vi "Rang wear off.vi"(8 "error in (no error)":errorcluster caption="错误输入（无错误）", 10 "字符串":string, 11 "Popup 输入":refnum<class "Popup.lvclass"> caption="DNL_LabVIEW Object in") -> (0 "error out":errorcluster caption="错误输出", 3 "Popup 输出":refnum<class "Popup.lvclass"> caption="DNL_LabVIEW Object out")   [LabVIEW 2017, in "Popup.lvclass"]
uses:
  Popup.lvclass
  Popup.lvclass/Popup.ctl
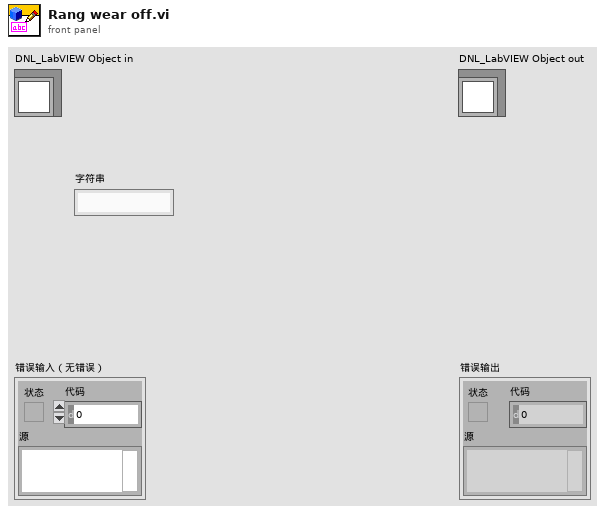
[diagram p1: front panel]
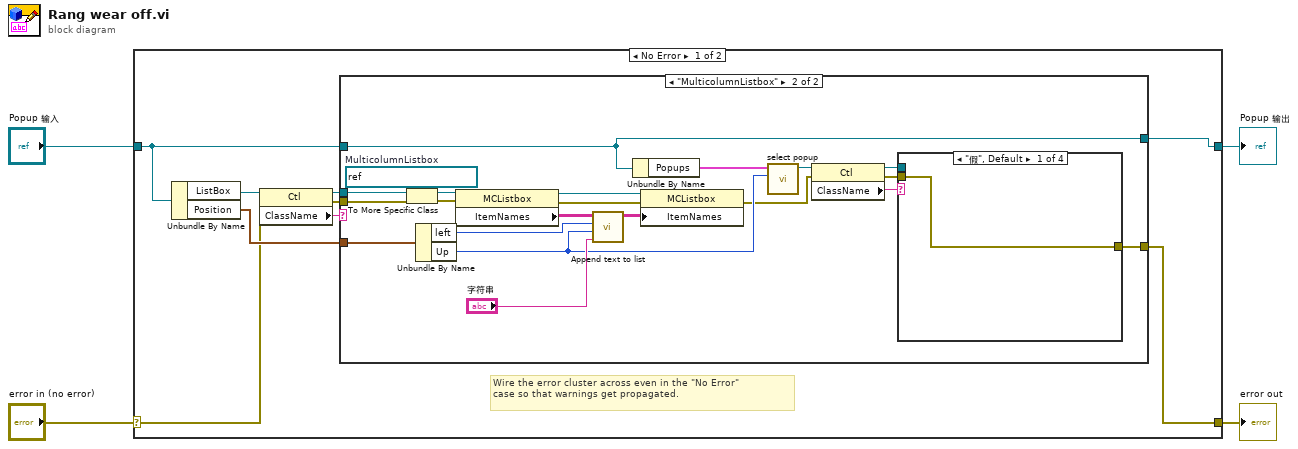
[diagram p0: block diagram]
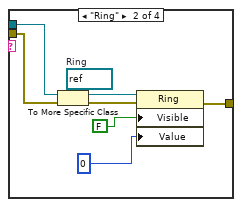
[diagram p3: hidden frame]
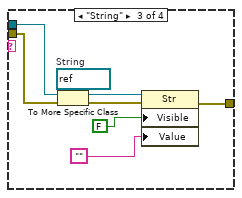
[diagram p4: hidden frame]
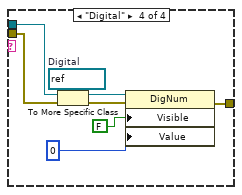
[diagram p5: hidden frame]
diagram:
  n1 = case shown="No Error" "error in (no error)" {
    selector: "error in (no error)" -> [w7 w63]
    tunnel: [w11 w63] -> w3
    tunnel: [w5 w62] -> w1
    tunnel: "Popup 输入" -> [w12 w62]
    frame No Error {
      # "Wire the error cluster across even in the \"No Error\"\ncase so that warnings get propagated."
      n2 = Unbundle By Name(w12) -> ("ListBox"=w10:refnum<vi>, "Position"=w13:cluster{"left":i32, "Up":i32})
      n3 = property class="Ctl"(reference=w10, error in=w7) -> (reference out=w9:refnum<vi>, error out=w8:errorcluster, "ClassName"=w6:string)
      n4 = case shown="\"MulticolumnListbox\"" w6 {
        tunnel: w13 -> [_ w33]
        tunnel: w12 -> [w14 w23]
        tunnel: [w15 w30] -> w11
        tunnel: w9 -> [_ w25]
        tunnel: w8 -> [w15 w24]
        tunnel: [w14 w23] -> w5
        frame "假", Default {
        }
        frame "MulticolumnListbox" {
          w36 = refnum<vi> refnum  # MulticolumnListbox
          n5 = To More Specific Class(target class=w36, reference=w25, error in=w24) -> (specific class reference=w35:refnum<vi>, error out=w34:errorcluster)
          n6 = Unbundle By Name(w33) -> ("left"=w27:i32, "Up"=w21:i32)
          n7 = property class="MCListbox"(reference=w35, error in=w34) -> (reference out=w32:refnum<vi>, error out=w31:errorcluster, "ItemNames"=w29:string[][])
          n8 = call "Append text to list.vi"("Text"="字符串", "Up"=w21, "Left"=w27, "List Text[]"=w29) -> ("List out[]"=w28:string[][])  [unwired: 7 in]
          n9 = Unbundle By Name(w23) -> ("Popups"=w22:cluster{"Referens":refnum<vi>, "Column":i32}[])
          n10 = property class="MCListbox"(reference=w32, error in=w31, "ItemNames"=w28) -> (error out=w19:errorcluster)  [unwired: 1 out]
          n11 = call "select popup.vi"("Column"=w21, "Popups"=w22) -> ("Ring输出"=w20:refnum<vi>)  [unwired: 9 in]
          n12 = property class="Ctl"(reference=w20, error in=w19) -> (reference out=w17:refnum<vi>, error out=w16:errorcluster, "ClassName"=w18:string)
          n13 = case shown="\"假\", Default" w18 {
            tunnel: [w37 w41 w49 w57] -> w30
            tunnel: w17 -> [_ w39 w48 w56]
            tunnel: w16 -> [w37 w38 w47 w55]
            frame "假", Default {
            }
            frame "Ring" {
              w45 = refnum<vi> refnum  # Ring
              n14 = To More Specific Class(target class=w45, reference=w39, error in=w38) -> (specific class reference=w44:refnum<vi>, error out=w43:errorcluster)
              n15 = property class="Ring"(reference=w44, error in=w43, "Visible"=FALSE, "Value"=u16 0) -> (error out=w41:errorcluster)  [unwired: 1 out]
            }
            frame "String" {
              w53 = refnum<vi> refnum  # String
              n16 = To More Specific Class(target class=w53, reference=w48, error in=w47) -> (specific class reference=w52:refnum<vi>, error out=w51:errorcluster)
              n17 = property class="Str"(reference=w52, error in=w51, "Visible"=FALSE, "Value"="") -> (error out=w49:errorcluster)  [unwired: 1 out]
            }
            frame "Digital" {
              w61 = refnum<vi> refnum  # Digital
              n18 = To More Specific Class(target class=w61, reference=w56, error in=w55) -> (specific class reference=w60:refnum<vi>, error out=w59:errorcluster)
              n19 = property class="DigNum"(reference=w60, error in=w59, "Visible"=FALSE, "Value"=0) -> (error out=w57:errorcluster)  [unwired: 1 out]
            }
          }
        }
      }
    }
    frame Error {
    }
  }
  "error out" <- w3
  "Popup 输出" <- w1
